vi "Anaylze Hand History.vi"() -> ()   [LabVIEW 2021]
panel:
  in  "reload":bool
  in  "stop":bool
  in  "Tab Control":T1(tab)
  out "Chip Stacks":dbl[][](graph)
  out "Card Map":T2(array[cluster]) {"Average Profit/Loss (BBs)" format="%#_3g"}
  out "Overall Profit/Loss (BBs)":dbl
  out "Total Hands":i32
  out "Shown Hands":string[](array[string])
  in  "Player":u16(ring) items=["Mark", "Jeff-T", "Jonathan-M", "Andrew", "Marty", "Ethan", "Ryan", "Michael-G", "Brian", "Jonathan-H", "Dennis"]
  out "Card Map (Shown)":T2(array[cluster]) {"Average Profit/Loss (BBs)" format="%#_3g"}
  out "Overall Profit/Loss (BBs, Shown)":dbl
  out "Total Hands (Shown)":i32
  in  "Date Mode":bool
  out "Waveform Graph":dbl[](graph)
  out "Mean":dbl
  out "All Hands":string[](array[string])
  # "SUITED"
  # "OFFSUIT"
  # "A"
  # "K"
  # "Q"
  # "J"
  # "T"
  # "9"
  # "8"
  # "7"
  # "6"
  # "5"
  # "4"
  # "3"
  # "2"
  # "2"
  # "3"
  # "4"
  # "5"
  # "6"
  # "7"
  # "8"
  # "9"
  # "T"
  # "J"
  # "Q"
  # "K"
  # "A"
  # "A"
  # "K"
  # "Q"
  # "J"
  # "T"
  # "9"
  # "8"
  # "7"
  # "6"
  # "5"
  # "4"
  # "3"
  # "2"
  # "2"
  # "3"
  # "4"
  # "5"
  # "6"
  # "7"
  # "8"
  # "9"
  # "T"
  # "J"
  # "Q"
  # "K"
  # "A"
  # "SUITED"
  # "OFFSUIT"
  # "A"
  # "K"
  # "Q"
  # "J"
  # "T"
  # "9"
  # "8"
  # "7"
  # "6"
  # "5"
  # "4"
  # "3"
  # "2"
  # "2"
  # "3"
  # "4"
  # "5"
  # "6"
  # "7"
  # "8"
  # "9"
  # "T"
  # "J"
  # "Q"
  # "K"
  # "A"
  # "A"
  # "K"
  # "Q"
  # "J"
  # "T"
  # "9"
  # "8"
  # "7"
  # "6"
  # "5"
  # "4"
  # "3"
  # "2"
  # "2"
  # "3"
  # "4"
  # "5"
  # "6"
  # "7"
  # "8"
  # "9"
  # "T"
  # "J"
  # "Q"
  # "K"
  # "A"
  # "STDDEVS"
  # "RAW"
  # "2"
  # "3"
  # "4"
  # "5"
  # "6"
  # "7"
  # "8"
  # "9"
  # "10"
  # "J"
  # "Q"
  # "K"
  # "A"
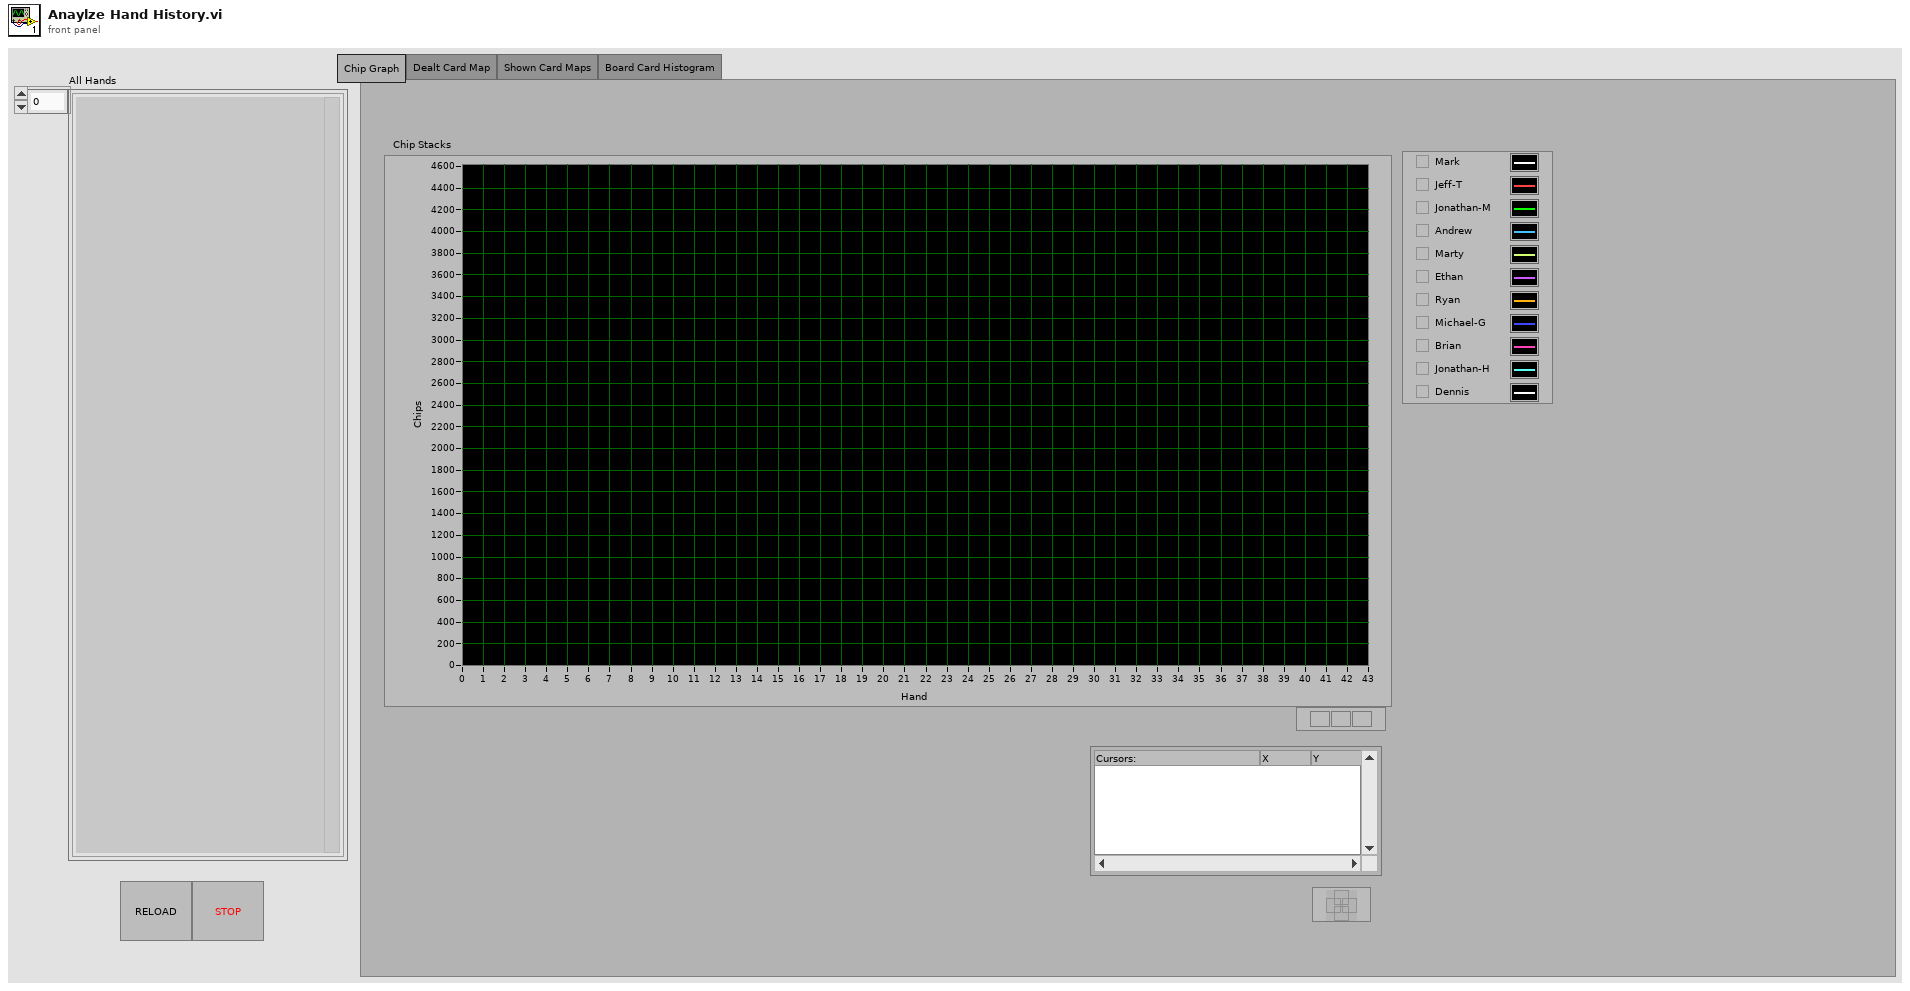
[diagram p1: front panel]
types:
  T1 = enum32{"Chip Graph", "Dealt Card Map", "Shown Card Maps", "Board Card Histogram"}
  T2 = cluster{"Hand Count":u16, "Average Profit/Loss (BBs)":dbl}[][]
  T3 = cluster{"Hand Count":u16, "Average Profit/Loss (BBs)":dbl}
  T4 = cluster{"Count":u16, "Profit/Loss (BBs)":dbl}[][]
  T5 = cluster{"Shown Hands":string[], "Card Map":cluster{"Hand Count":u16, "Average Profit/Loss (BBs)":dbl}[][], "Total Hands":i32, "Overall Profit Loss (BBs)":dbl}
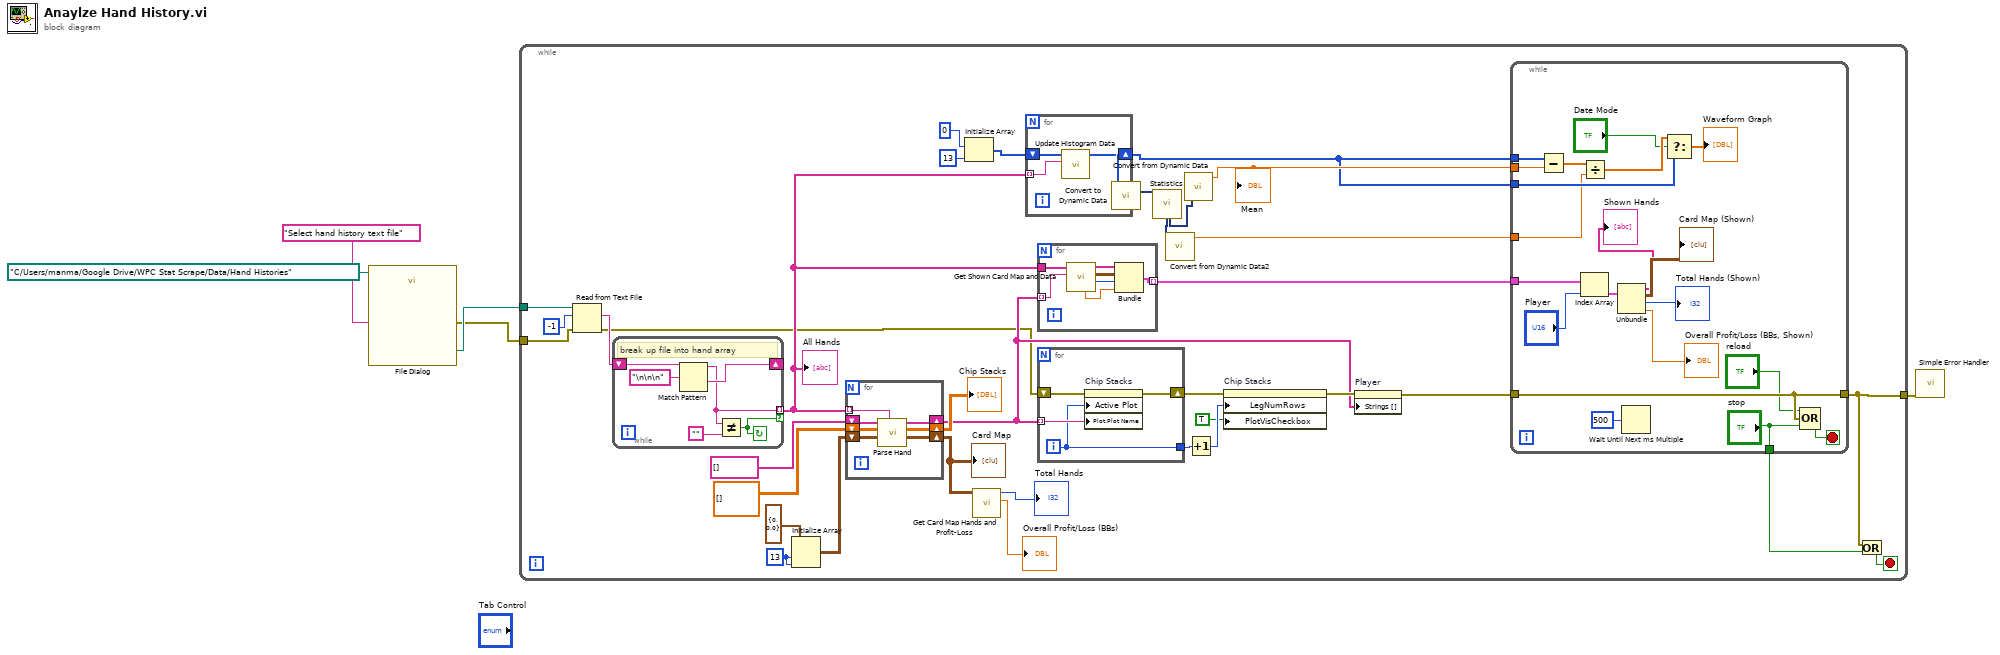
[diagram p0: block diagram]
diagram:
  n1 = call "File Dialog"("start path"=path "C:/Users/manma/Google Drive/WPC Stat Scrape/Data/Hand Histories", "prompt"="Select hand history text file" ("prompt (Open existing file)")) -> ("selected path"=w2:path, "error out"=w1:errorcluster)  [unwired: 10 in, 2 out]
  n2 = while {
    tunnel: [w18] -> w5
    tunnel: w2 -> [w15]
    tunnel: w1 -> [w14]
    stop <- w16 stop-if-true
    w30 = 13 ("dimension size")
    n3 = Read from Text File(file (use dialog)=w15, count=-1, error in=w14) -> (text=w39:string, error out=w13:errorcluster)  [unwired: 1 in, 2 out]
    n4 = while {
      shift-right: [w86] -> _
      shift-left: w39 -> [w87]
      tunnel: [w84] -> w22 mode=indexing if=w82
      stop <- w82 continue-if-true
      # "break up file into hand array"
      n5 = Match Pattern(string=w87, regular expression="\n\n\n") -> (before substring=w84:string, after substring=w86:string)  [unwired: 1 in, 2 out]
      n6 = Not Equal?(x=w84, y="") -> (x != y?=w82:bool)
    }
    "All Hands" <- w22
    n7 = Initialize Array(T3 {"Hand Count"=0, "Average Profit/Loss (BBs)"=0.0} ("Cluster"), w30, w30) -> (w29:T2)
    n8 = for {
      tunnel: w22 -> [w77] mode=indexing
      shift-right: [w80] -> w24
      shift-left: string[] [] -> [w81]
      shift-right: [w78] -> w33
      shift-left: dbl[][] [] -> [w79]
      shift-right: [w75] -> w28
      shift-left: w29 -> [w76]
      n9 = call "Parse Hand.vi"("Hand History String"=w77, "Card Map In"=w76, "Chip Stacks"=w79, "Player Names"=w81) -> ("Card Map Out"=w75:T4, "Chip Stacks Out"=w78:dbl[][], "Player Names Out"=w80:string[])  [unwired: 5 in]
    }
    "Chip Stacks" <- w33
    "Card Map" <- w28
    n10 = Initialize Array(0, 13 ("dimension size")) -> (w21:i32[])
    n11 = call "Get Card Map Hands and Profit-Loss.vi"("Card Map In"=w28) -> ("Profit/Loss (BBs)"=→"Overall Profit/Loss (BBs)":dbl, "Total Hands"=→"Total Hands":i32)  [unwired: 9 in]
    n12 = for {
      tunnel: w22 -> [w41] mode=indexing
      shift-right: [w42] -> w7
      shift-left: w21 -> [w43]
      n13 = call "Update Histogram Data.vi"("Hand String"=w41, "Histogram In"=w43) -> ("Histogram Out"=w42:i32[])  [unwired: 9 in]
    }
    n14 = for {
      tunnel: w24 -> [w74] mode=indexing
      shift-right: [w72] -> w34
      shift-left: w13 -> [w73]
      tunnel: [w71] -> w37
      i -> [w71]
      n15 = property on="Chip Stacks" class="WFGraph (strict)"(error in=w73, "Active Plot"=w71, "Plot.Plot Name"=w74) -> (error out=w72:errorcluster)  [unwired: 1 in, 1 out]
    }
    n16 = for {
      tunnel: w22 -> [w70]
      tunnel: w24 -> [w69] mode=indexing
      tunnel: [w65] -> w23 mode=indexing
      n17 = call "Get Shown Card Map and Data.vi"("Player"=w69, "Hand Array"=w70) -> ("Total Hands"=w67:i32, "Card Map"=w68:T2, "Shown Hands"=w64:string[], "Overall Profit Loss (BBs)"=w66:dbl)  [unwired: 6 in]
      n18 = Bundle("Shown Hands"=w64, "Card Map"=w68, "Total Hands"=w67, "Overall Profit Loss (BBs)"=w66) -> (w65:T5)  [unwired: 1 in]
    }
    n19 = call "Convert to Dynamic Data"("Array"=w7) -> ("Dynamic Data Type"=w11:dynamicdata)  [unwired: 3 in]
    n20 = call "Statistics"("Signals"=w11) -> ("Standard Dev"=w9:dynamicdata, "Arithmetic Mean"=w10:dynamicdata)  [unwired: 24 in, 1 out]
    n21 = call "Convert from Dynamic Data2"("Dynamic Data Type"=w9) -> ("Scalar"=w6:dbl)  [unwired: 3 in]
    n22 = call "Convert from Dynamic Data"("Dynamic Data Type"=w10) -> ("Scalar"=w8:dbl)  [unwired: 3 in]
    "Mean" <- w8
    n23 = Increment(x=w37) -> (x+1=w36:i32)
    n24 = property on="Chip Stacks" class="WFGraph (strict)"(error in=w34, "LegNumRows"=w36, "PlotVisCheckbox"=TRUE ("Legend:Plot Visibility Checkbox Visible")) -> (error out=w25:errorcluster)  [unwired: 1 in, 1 out]
    n25 = property on="Player" class="Ring (strict)"(error in=w25, "Strings []"=w24) -> (error out=w12:errorcluster)  [unwired: 1 in, 1 out]
    n26 = while {
      tunnel: w12 -> [w62]
      tunnel: [w62] -> w18
      tunnel: w23 -> [w61]
      tunnel: ["stop"] -> w17
      tunnel: w7 -> [w47]
      tunnel: w8 -> [w46]
      tunnel: w7 -> [w45]
      tunnel: w6 -> [w44]
      stop <- w63 stop-if-true
      n27 = Subtract(x=w45, y=w46) -> (x-y=w48:dbl[])
      n28 = Index Array(array=w61, index="Player") -> (element=w59:T5)
      n29 = Divide(x=w48, y=w44) -> (x/y=w50:dbl[])
      n30 = Unbundle(w59) -> ("Shown Hands"=→"Shown Hands":string[], "Card Map"=→"Card Map (Shown)":T2, "Total Hands"=→"Total Hands (Shown)":i32, "Overall Profit Loss (BBs)"=→"Overall Profit/Loss (BBs, Shown)":dbl)
      n31 = Wait Until Next ms Multiple(millisecond multiple=u32 500) -> ()  [unwired: 1 out]
      n32 = Select(t=w50, s="Date Mode", f=w47) -> (s? t:f=→"Waveform Graph":dbl[])
      n33 = Compound Arithmetic op=OR("reload", w62, "stop") -> (w63:bool)
    }
    n34 = Or(x=w18, y=w17) -> (x .or. y?=w16:bool)
  }
  n35 = call <vilib>:"Simple Error Handler.vi"("error in (no error)"=w5) -> ()  [unwired: 4 in, 5 out]
